vi "zad9.vi"() -> ()   [LabVIEW 2025]
uses:
  state.ctl
panel:
  in  "Stop":bool
  in  "reset record":bool
  out "Pressed numbers":string
  in  "Button 3":bool
  in  "Button 0":bool
  in  "Button 2":bool
  in  "Button 1":bool
  in  "Button 6":bool
  in  "Button 5":bool
  in  "Button 4":bool
  in  "Button 9":bool
  in  "Button 8":bool
  in  "Button 7":bool
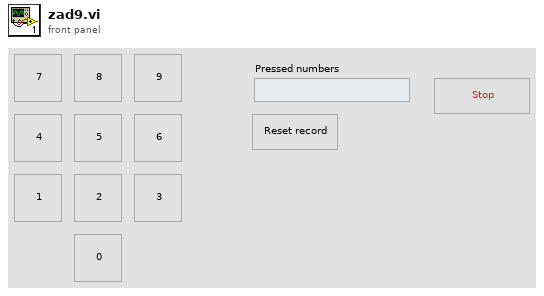
[diagram p1: front panel]
types:
  T1 = typedef "state.ctl" = enum16{"Type_number", "Show_number", "Reset_record", "Stop"}
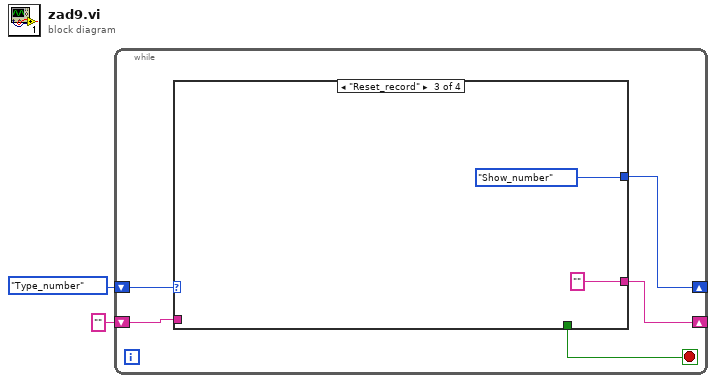
[diagram p0: block diagram]
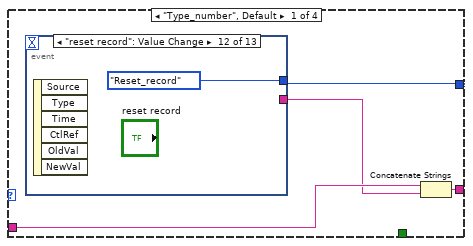
[diagram p2: hidden frame]
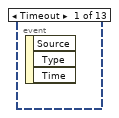
[diagram p3: hidden frame]
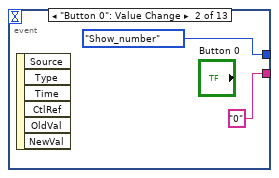
[diagram p4: hidden frame]
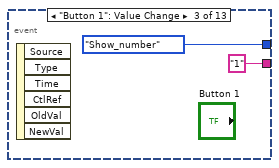
[diagram p5: hidden frame]
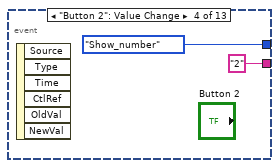
[diagram p6: hidden frame]
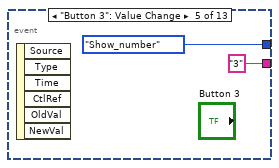
[diagram p7: hidden frame]
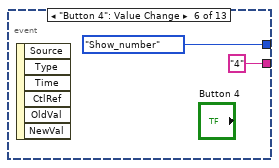
[diagram p8: hidden frame]
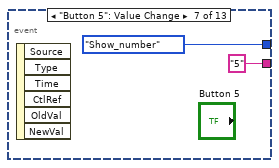
[diagram p9: hidden frame]
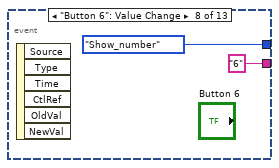
[diagram p10: hidden frame]
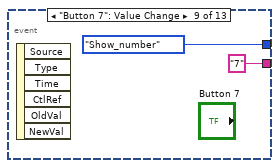
[diagram p11: hidden frame]
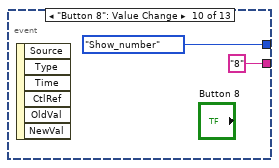
[diagram p12: hidden frame]
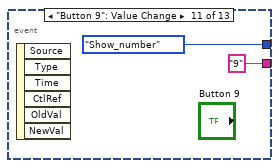
[diagram p13: hidden frame]
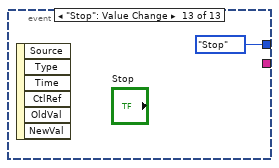
[diagram p14: hidden frame]
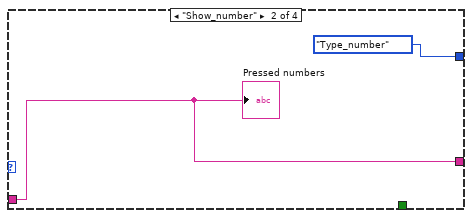
[diagram p15: hidden frame]
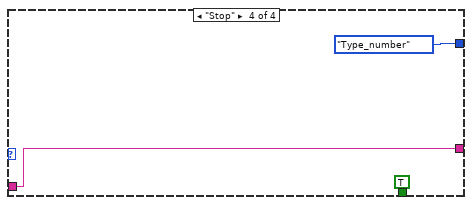
[diagram p16: hidden frame]
diagram:
  n1 = while {
    shift-right: [w6] -> _
    shift-left: state."Type_number" -> [w7]
    shift-right: [w4] -> _
    shift-left: "" -> [w5]
    stop <- w3 stop-if-true
    n2 = case shown="\"Reset_record\"" w7 {
      tunnel: [w11 state."Type_number" state."Show_number" state."Type_number"] -> w6
      tunnel: w5 -> [w10 w35 _ w39]
      tunnel: [w8 w35 "" w39] -> w4
      tunnel: [_ _ _ TRUE] -> w3
      frame "Type_number", Default {
        n3 = event shown="[11] \"reset record\": Value Change" {
          selector: _ -> [_ _ _ _ _ _ _ _ _ _ _ _ _]
          dyn-events: _ -> [_ _ _ _ _ _ _ _ _ _ _ _ _]
          timeout: _ -> [_ _ _ _ _ _ _ _ _ _ _ _ _]
          tunnel: [_ state."Show_number" state."Show_number" state."Show_number" state."Show_number" state."Show_number" state."Show_number" state."Show_number" state."Show_number" state."Show_number" state."Show_number" state."Reset_record" state."Stop"] -> w11
          tunnel: [_ "0" "1" "2" "3" "4" "5" "6" "7" "8" "9" _ _] -> w9
          event Timeout {
            n4 = event-data() -> ()  [unwired: 1 in, 3 out]
          }
          event "Button 0": Value Change {
            n5 = event-data() -> ()  [unwired: 1 in, 6 out]
          }
          event "Button 1": Value Change {
            n6 = event-data() -> ()  [unwired: 1 in, 6 out]
          }
          event "Button 2": Value Change {
            n7 = event-data() -> ()  [unwired: 1 in, 6 out]
          }
          event "Button 3": Value Change {
            n8 = event-data() -> ()  [unwired: 1 in, 6 out]
          }
          event "Button 4": Value Change {
            n9 = event-data() -> ()  [unwired: 1 in, 6 out]
          }
          event "Button 5": Value Change {
            n10 = event-data() -> ()  [unwired: 1 in, 6 out]
          }
          event "Button 6": Value Change {
            n11 = event-data() -> ()  [unwired: 1 in, 6 out]
          }
          event "Button 7": Value Change {
            n12 = event-data() -> ()  [unwired: 1 in, 6 out]
          }
          event "Button 8": Value Change {
            n13 = event-data() -> ()  [unwired: 1 in, 6 out]
          }
          event "Button 9": Value Change {
            n14 = event-data() -> ()  [unwired: 1 in, 6 out]
          }
          event "reset record": Value Change {
            n15 = event-data() -> ()  [unwired: 1 in, 6 out]
          }
          event "Stop": Value Change {
            n16 = event-data() -> ()  [unwired: 1 in, 6 out]
          }
        }
        n17 = Concatenate Strings(w10, w9) -> (w8:string)
      }
      frame "Show_number" {
        "Pressed numbers" <- w35
      }
      frame "Reset_record" {
      }
      frame "Stop" {
      }
    }
  }
